vi "Handle Error.vi"(8 "error in (no error)":errorcluster, 11 "Model Base in":refnum<class "Model Base.lvclass">) -> (0 "error out":errorcluster, 2 "stop actor?":bool=TRUE, 3 "Model Base out":refnum<class "Model Base.lvclass">)   [LabVIEW 2023, in "Model Base.lvlib" / "Model Base.lvclass"]
doc: "(<B>Filename</B>: Actor Framework.lvlib:Actor.lvclass:Handle Error.vi)\n\nDefines how the actor handles an error that occurred while processing a message. By default, this method does nothing except stop the actor."
uses:
  Model Base.lvclass
  <vilib>/ActorFramework/Actor/Actor.lvclass
  Model Base.lvclass/Model Base.ctl
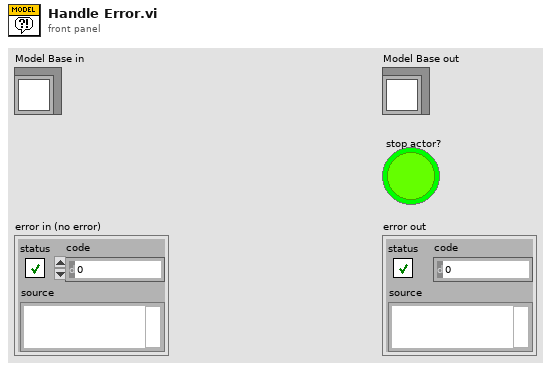
[diagram p1: front panel]
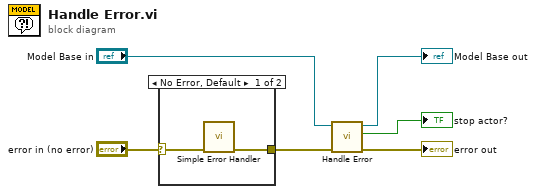
[diagram p0: block diagram]
diagram:
  n1 = case shown="No Error, Default" "error in (no error)" {
    selector: "error in (no error)" -> [w8 w9]
    tunnel: [w7 w9] -> w1
    frame No Error {
      n2 = call <vilib>:"Simple Error Handler.vi"("error in (no error)"=w8) -> ("error out"=w7:errorcluster)  [unwired: 4 in, 4 out]
    }
    frame Error {
    }
  }
  n3 = call-parent "Handle Error.vi"("error in (no error)"=w1, "Actor in"="Model Base in") -> ("error out"=→"error out":errorcluster, "stop actor?"=→"stop actor?":bool, "Actor out"=→"Model Base out":refnum<class "Model Base.lvclass">)  [unwired: 7 in]
